vi "Send Usb Data.vi"(8 "error in (no error)":errorcluster, 10 "Length":u32, 11 "Buffer":u8[](array[numeric])) -> (0 "error out":errorcluster)   [LabVIEW 2015, in "TPVG_DLL.lvlib"]
doc: "This function is used to send a information on the USB link\nusing the packet protocol\n\n\nDWORD CLASS_DECLSPEC SendUsbData( BYTE*, DWORD );"
uses:
  TPVG_DLL.lvlib
  TPVG_DLL.dll
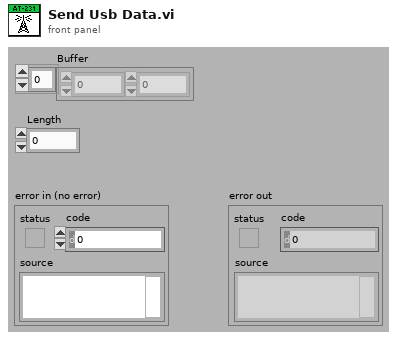
[diagram p1: front panel]
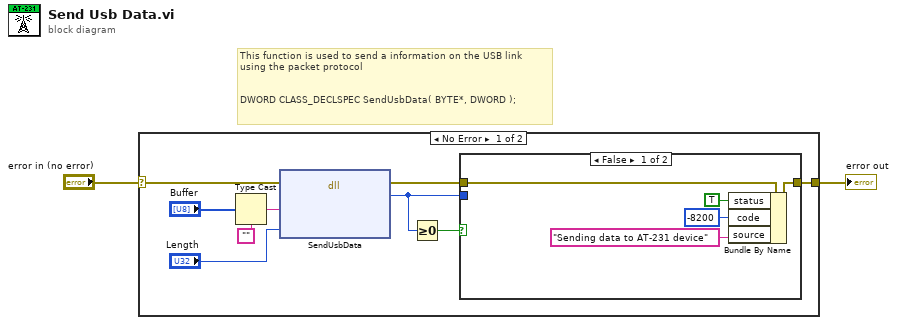
[diagram p0: block diagram]
diagram:
  # "This function is used to send a information on the USB link\nusing the packet protocol\n\n\nDWORD CLASS_DECLSPEC SendUsbData( BYTE*, DWORD );"
  n1 = case shown="No Error" "error in (no error)" {
    selector: "error in (no error)" -> [w7 w18]
    tunnel: [w3 w18] -> w2
    frame No Error {
      n2 = Type Cast(type="", x="Buffer") -> (*(type *) &x=w9:string)
      n3 = dll-call lib="\\\\Mac\\Home/Desktop/imt_test_app 28-06-2012/TPVG_DLL.dll" fn="SendUsbData"(error in=w7, "Buffer"=w9, "Length"="Length") -> (error out=w5:errorcluster, "Return"=w4:u32)  [unwired: 4 in, 1 out]
      n4 = Greater Or Equal To 0?(x=w4) -> (x >= 0?=w6:bool)
      n5 = case shown="False" w6 {
        tunnel: w5 -> [w16 w17]
        tunnel: w4 -> [_ _]
        tunnel: [w15 w17] -> w3
        frame False {
          n6 = Bundle By Name(cluster=w16, "status"=TRUE, "code"=-8200, "source"="Sending data to AT-231 device") -> (w15:errorcluster)
        }
        frame True {
        }
      }
    }
    frame Error {
    }
  }
  "error out" <- w2
